vi "Create Queue.vi"(6 "FIFO":bool, 8 "error in (no error)":errorcluster, 9 "Region":T1, 10 "Name":string, 11 "AWS Credentials":T2) -> (0 "error out":errorcluster, 3 "SQS":refnum<class "Queue.lvclass">)   [LabVIEW 2015, in "NI_AWS_SQS.lvlib" / "Queue.lvclass"]
uses:
  Queue.lvclass
  Core/HTTP Request/AWS Credentials.ctl
  Core/HTTP Request/Region.ctl
  Core/HTTP Request/Request Options.ctl
  Core/HTTP Request/Name Value Pair.ctl
  Core/HTTP Request/HTTP Request.lvclass/HTTP Request.ctl
  Queue.lvclass/Queue.ctl
  Core/HTTP Request/Write Credentials.vi
  Core/HTTP Request/Write Region.vi
  Core/HTTP Request/Write Service.vi
  Core/HTTP Request/Write Verify Server.vi
  Write FIFO.vi
  Write Account Number.vi
  Write Name.vi
  Write URL.vi
  <vilib>/Utility/error.llb/Error Cluster From Error Code.vi
  <vilib>/ErrorRing/Error Ring.xnode
  Core/HTTP Request/HTTP Request.lvclass
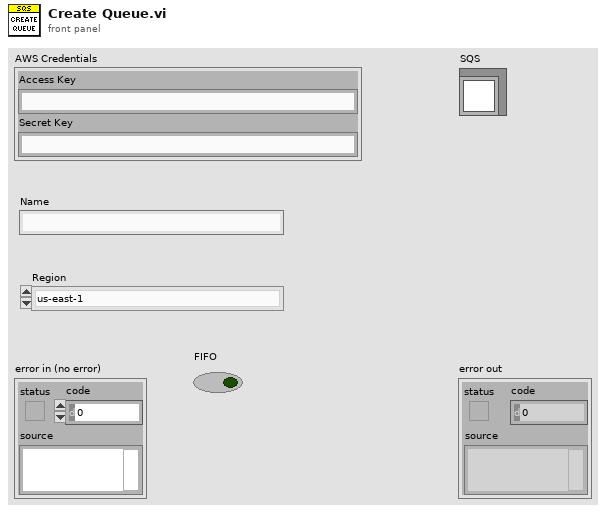
[diagram p1: front panel]
types:
  T1 = typedef "NI_AWS_Core.lvlib/HTTP Request.lvclass/Region.ctl" = enum16{"us-east-1", "us-east-2", "us-west-1", "us-west-2", "ap-northeast-1", "ap-northeast-2", "ap-southeast-1", "ap-southeast-2", "ca-central-1", "eu-central-1", "eu-west-1", "eu-west-2", "sa-east-1"}
  T2 = typedef "NI_AWS_Core.lvlib/HTTP Request.lvclass/AWS Credentials.ctl" = cluster{"Access Key":string, "Secret Key":string}
  T3 = typedef "NI_AWS_Core.lvlib/HTTP Request.lvclass/Name Value Pair.ctl" = cluster{"name":string, "value":string}
  T4 = typedef "NI_AWS_Core.lvlib/HTTP Request.lvclass/Request Options.ctl" = cluster{"request headers":T3[], "request parameters":T3[], "request body":string}
  T5 = typedef "NI_AWS_Core.lvlib/HTTP Request.lvclass/Response.ctl" = cluster{"Headers":string, "Body":string}
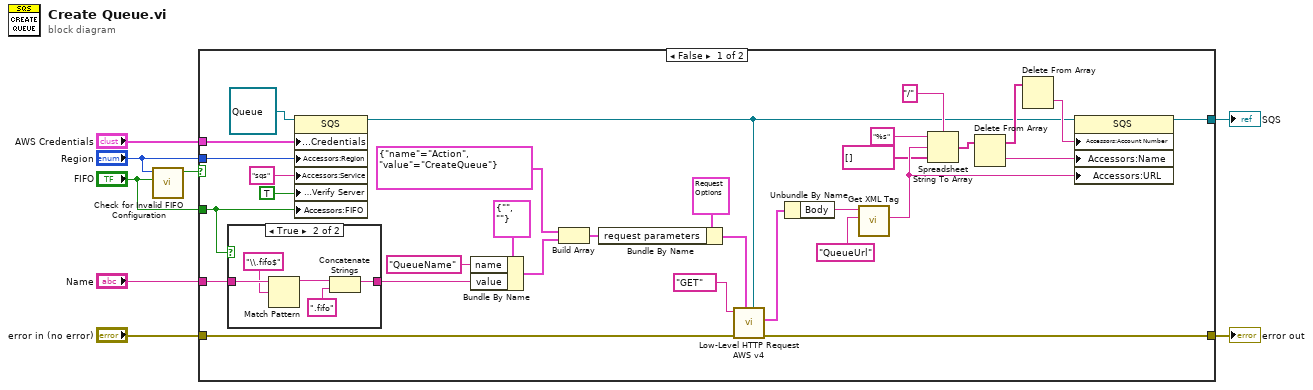
[diagram p0: block diagram]
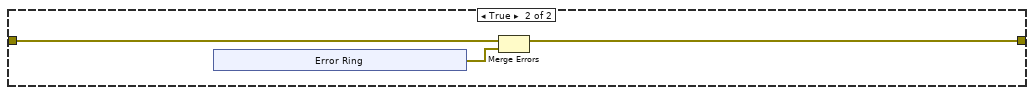
[diagram p3: hidden frame]
diagram:
  n1 = call "Check for Invalid FIFO Configuration.vi"("Desired FIFO"="FIFO", "Region"="Region") -> ("Invalid FIFO Configuration"=w2:bool)  [unwired: 9 in]
  n2 = case shown="False" w2 {
    tunnel: "AWS Credentials" -> [w36 _]
    tunnel: [w32 w47] -> w7
    tunnel: "error in (no error)" -> [w31 w48]
    tunnel: [w18 _] -> w5
    tunnel: "Name" -> [w11 _]
    tunnel: "Region" -> [w12 _]
    tunnel: "FIFO" -> [w9 _]
    frame False {
      n3 = case shown="True" w9 {
        tunnel: w11 -> [w40 w45]
        tunnel: [w40 w42] -> w10
        frame False {
        }
        frame True {
          n4 = Match Pattern(string=w45, regular expression="\\.fifo$") -> (before substring=w43:string)  [unwired: 1 in, 3 out]
          n5 = Concatenate Strings(w43, ".fifo") -> (w42:string)
        }
      }
      n6 = property class="SQS"(reference=refnum<class "Queue.lvclass"> refnum ("NI_SQS.lvlib:SQS"), "Accessors:Credentials"=w36, "Accessors:Region"=w12, "Accessors:Service"="sqs" ("Service"), "Accessors:Verify Server"=TRUE ("Verify Server"), "Accessors:FIFO"=w9) -> (reference out=w19:refnum<class "Queue.lvclass">)  [unwired: 1 in, 1 out]
      n7 = Bundle By Name(cluster=T3 {"name"="", "value"=""} ("element"), "name"="QueueName", "value"=w10) -> (w13:T3)
      n8 = Build Array(T3 {"name"="Action", "value"="CreateQueue"} ("Name Value Pair"), w13) -> (w17:T3[])
      n9 = Bundle By Name(cluster=T4 {"request headers"=[], "request parameters"=[{"name"="Action", "value"="ListQueues"}], "request body"=""} ("Request Options"), "request parameters"=w17) -> (w35:T4)
      n10 = call "Low-Level HTTP Request AWS v4.vi"("AWS Core"=w19, "Request Options"=w35, "error in (no error)"=w31, "HTTP-Verb"="GET") -> ("error out"=w32:errorcluster, "Response"=w21:T5)  [unwired: 5 in, 1 out]
      n11 = Unbundle By Name(w21) -> ("Body"=w20:string)
      n12 = call "Get XML Tag.vi"("Tag name"="QueueUrl", "XML String in"=w20) -> ("Tag value"=w29:string)  [unwired: 5 in, 4 out]
      n13 = Spreadsheet String To Array(delimiter (Tab)="/", format string="%s", spreadsheet string=w29, array type (2D Dbl)=string[] []) -> (array=w25:string[])
      n14 = Delete From Array(array=w25) -> (deleted portion=w24:string, array with subset deleted=w23:string[])  [unwired: 2 in]
      n15 = Delete From Array(array=w23) -> (deleted portion=w22:string)  [unwired: 2 in, 1 out]
      n16 = property class="SQS"(reference=w19, "Accessors:Account Number"=w22, "Accessors:Name"=w24, "Accessors:URL"=w29) -> (reference out=w18:refnum<class "Queue.lvclass">)  [unwired: 1 in, 1 out]
    }
    frame True {
      n17 = xnode "Error Ring"() -> ("error out"=w46:errorcluster)
      n18 = Merge Errors(w48, w46) -> (w47:errorcluster)
    }
  }
  "error out" <- w7
  "SQS" <- w5
